vi "Global - Device Type.vi"() -> ()   [LabVIEW 2019]
panel:
  in  "Datalog":bool[](array[boolean])
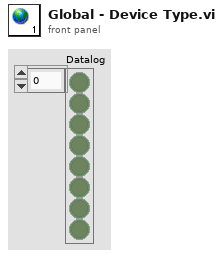
[diagram p1: front panel]
diagram:
